vi "Actor Core.vi"(8 "error in":errorcluster, 11 "Nested in":refnum<class "Nested.lvclass">) -> (0 "error out":errorcluster, 3 "Actor out":refnum<class "Actor.lvclass">)   [LabVIEW 2020, in "Nested.lvlib" / "Nested.lvclass"]
doc: "(<B>Filename</B>: Actor Framework.lvlib:Actor.lvclass:Actor Core.vi)\n\nReceives messages to the actor, reacts to them, and initiates any error handling that may shut the actor down.\n\nDescendant classes may override this VI to append parallel tasks for the actor to complete while it handles messages. Overrides use the Call Parent Class Method node."
uses:
  Nested.lvclass
  <vilib>/ActorFramework/Actor/Actor.lvclass
  Nested.lvclass/Nested.ctl
  <vilib>/ActorFramework/Message Enqueuer/Message Enqueuer.lvclass/Message Enqueuer.ctl
  Caller/Caller Messages/PopUP Msg/PopUP Msg.lvclass/PopUP Msg.ctl
  Caller/Caller Messages/UpdateMessage Msg/UpdateMessage Msg.lvclass/UpdateMessage Msg.ctl
  <vilib>/ActorFramework/Message Enqueuer/Enqueue.vi
  <vilib>/ActorFramework/Stop Msg/Stop Msg.lvclass
  C:/Program Files/National Instruments/LabVIEW 2020/vi.lib/ActorFramework/Message/Message.lvclass
  Nested Messages/GenerateSin Msg/GenerateSin Msg.lvclass
  Nested Messages/Error state Msg/Error state Msg.lvclass
  Caller/Caller Messages/PopUP Msg/PopUP Msg.lvclass
  Caller/Caller Messages/UpdateMessage Msg/UpdateMessage Msg.lvclass
  <vilib>/ActorFramework/Message Priority Queue/Priority Enqueue.vi
panel:
  in  "Btn_ Send _Caller":bool
  in  "Btn_Error":bool
  out "Waveform Chart":dbl(graph)
  # "Nested"
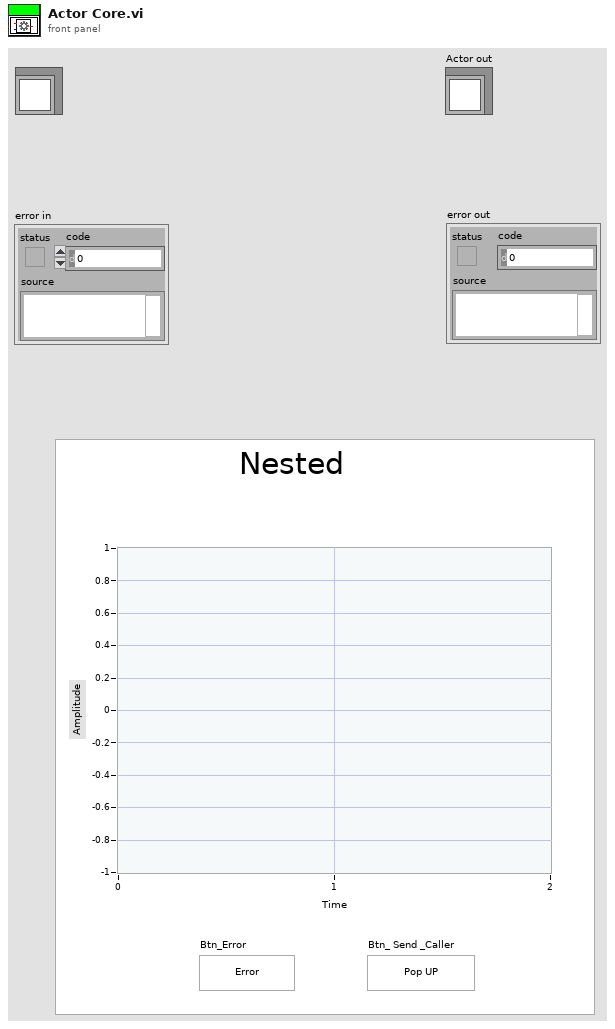
[diagram p1: front panel]
types:
  T1 = cluster{"Quit":refnum<user-event>, "WaveformDisplay":refnum<user-event>}
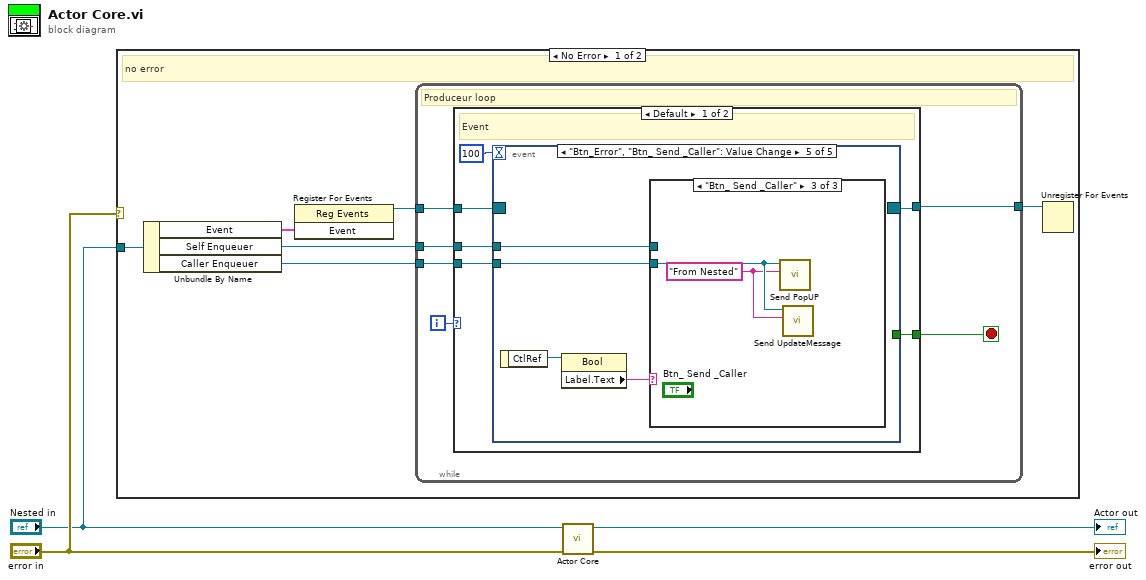
[diagram p0: block diagram]
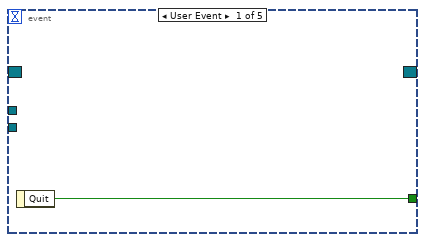
[diagram p2: hidden frame]
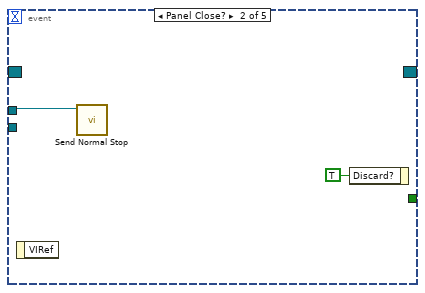
[diagram p3: hidden frame]
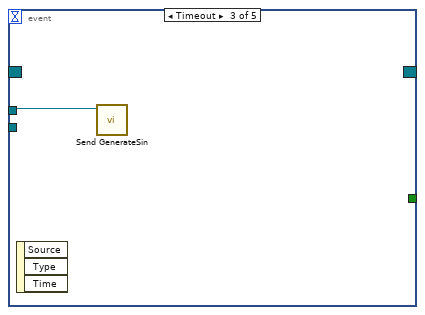
[diagram p4: hidden frame]
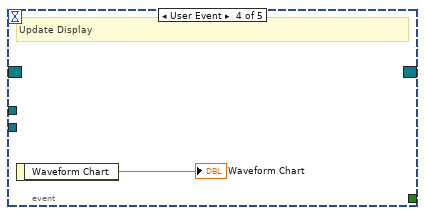
[diagram p5: hidden frame]
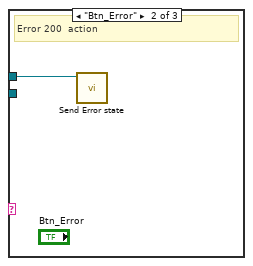
[diagram p7: hidden frame]
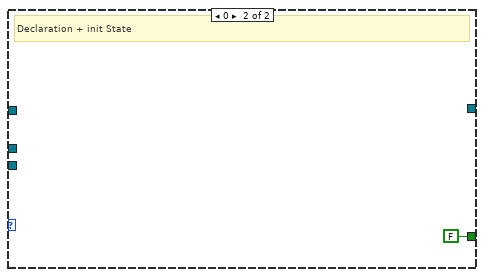
[diagram p8: hidden frame]
diagram:
  n1 = case shown="No Error" "error in" {
    tunnel: "Nested in" -> [w10 _]
    frame No Error {
      # "no error"
      n2 = Unbundle By Name(w10) -> ("Event"=w9:T1, "Self Enqueuer"=w6:refnum<class "Message Enqueuer.lvclass">, "Caller Enqueuer"=w5:refnum<class "Message Enqueuer.lvclass">)
      n3 = register-events(w9) -> (reference out=w8:refnum<event-registration>)  [unwired: 2 in, 1 out]
      n4 = while {
        tunnel: w8 -> [w14]
        tunnel: [w13] -> w7
        tunnel: w6 -> [w12]
        tunnel: w5 -> [w11]
        i -> [w16]
        stop <- w15 stop-if-true
        # "Produceur loop"
        n5 = case shown="Default" w16 {
          tunnel: [w20 FALSE] -> w15
          tunnel: w14 -> [w22 _]
          tunnel: [w21 _] -> w13
          tunnel: w12 -> [w19 _]
          tunnel: w11 -> [w17 _]
          frame Default {
            # "Event"
            n6 = event shown="[4] \"Btn_Error\", \"Btn_ Send _Caller\": Value Change" {
              selector: w22 -> [_ _ _ _ _]
              dyn-events: [_ _ _ _ _] -> w21
              timeout: 100 -> [_ _ _ _ _]
              tunnel: [w23 _ _ _ _] -> w20
              tunnel: w19 -> [_ w24 w26 _ w29]
              tunnel: w17 -> [_ _ _ _ w28]
              event User Event {
                n7 = event-data() -> ("Quit"=w23:bool)  [unwired: 1 in]
              }
              event Panel Close? {
                n8 = event-data() -> ()  [unwired: 1 in, 1 out]
                n9 = call <vilib>:"Send Normal Stop.vi"("Message Enqueuer"=w24) -> ()  [unwired: 10 in, 1 out]
                n10 = event-data("Discard?"=TRUE) -> ()  [unwired: 1 in, 1 out]
              }
              event Timeout {
                n11 = event-data() -> ()  [unwired: 1 in, 3 out]
                n12 = call "Send GenerateSin.vi"("Message Enqueuer"=w26) -> ()  [unwired: 9 in, 2 out]
              }
              event User Event {
                # "Update Display"
                n13 = event-data() -> ("Waveform Chart"=→"Waveform Chart":dbl)  [unwired: 1 in]
              }
              event "Btn_Error", "Btn_ Send _Caller": Value Change {
                n14 = event-data() -> ("CtlRef"=w31:refnum<vi>)  [unwired: 1 in]
                n15 = property class="Bool"(reference=w31) -> ("Label.Text"=w30:string)  [unwired: 1 in, 2 out]
                n16 = case shown="\"Btn_ Send _Caller\"" w30 {
                  tunnel: w29 -> [_ w32 _]
                  tunnel: w28 -> [_ _ w34]
                  frame Default {
                    # "Do nothing"
                  }
                  frame "Btn_Error" {
                    # "Error 200  action"
                    n17 = call "Send Error state.vi"("Message Enqueuer"=w32) -> ()  [unwired: 9 in, 2 out]
                  }
                  frame "Btn_ Send _Caller" {
                    w33 = "From Nested" ("PopUP")
                    n18 = call "Send PopUP.vi"("PopUP"=w33, "Message Enqueuer"=w34) -> ()  [unwired: 8 in, 2 out]
                    n19 = call "Send UpdateMessage.vi"("Message"=w33, "Message Enqueuer"=w34) -> ()  [unwired: 8 in, 2 out]
                  }
                }
              }
            }
          }
          frame 0 {
            # "Declaration + init State"
          }
        }
      }
      n20 = Unregister For Events(event registration refnum=w7) -> ()  [unwired: 1 in, 1 out]
    }
    frame Error {
    }
  }
  n21 = call-parent "Actor Core.vi"("error in"="error in", "Actor in"="Nested in") -> ("error out"=→"error out":errorcluster, "Actor out"=→"Actor out":refnum<class "Actor.lvclass">)  [unwired: 8 in]
